vi "Positions.vi"() -> ()   [LabVIEW 2019]
uses:
  <vilib>/Rock Robotics/WPI/Solenoid/WPI_SolenoidValue.ctl
panel:
  in  "CLIMBER_UP":dbl
  in  "SHOOTER_SPEED":dbl
  in  "SHOOTER_ANGLE_MIN":dbl
  in  "SHOOTER_ANGLE_MAX":dbl
  in  "TURRET_MIN":dbl
  in  "TURRET_MAX":dbl
  in  "LOW_GEAR":T1
  in  "HIGH_GEAR":T1
  in  "INTAKE_DOWN":T1
  in  "INTAKE_UP":T1
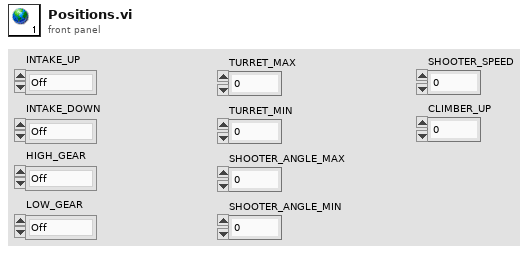
[diagram p1: front panel]
types:
  T1 = typedef "WPI_SolenoidValue.ctl" = enum16{"Off", "On", "Forward", "Reverse"}
diagram:
